vi "Refresh Players.vi"(11 "Dashboard":refnum<vi>) -> ()   [LabVIEW 2015, in "SB SubVIs.lvlib"]
uses:
  SB SubVIs.lvlib
  Type Defs/Dashboard.ctl
  Type Defs/Add Player.ctl
  Square/Square.lvclass
  Globals (private).vi
  Type Defs/SB Type Defs.lvlib
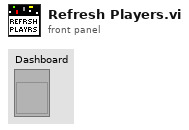
[diagram p1: front panel]
types:
  T1 = cluster{"Square out":refnum<class "Square.lvclass">, "Name":string, "Victory Speech":string}
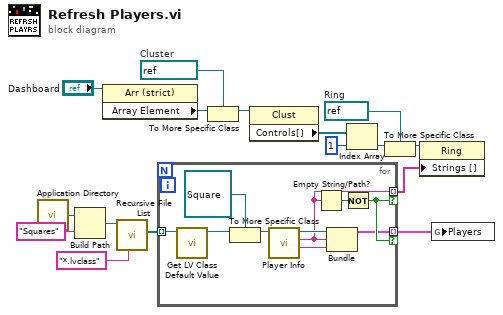
[diagram p0: block diagram]
diagram:
  w4 = refnum<vi> refnum  # Ring
  w9 = refnum<vi> refnum  # Cluster
  n1 = call <vilib>:"Application Directory.vi"() -> ("Application Directory"=w13:path)
  n2 = Build Path(base path=w13, name or relative path="Squares") -> (appended path=w11:path)
  n3 = property class="Arr (strict)"(reference="Dashboard") -> ("Array Element"=w10:refnum<vi>)  [unwired: 1 in, 2 out]
  n4 = call <vilib>:"Recursive File List.vi"("pattern"="*.lvclass", "Folder Path"=w11) -> ("All Files in Dir"=w15:path[])  [unwired: 5 in, 4 out]
  n5 = for {
    tunnel: w15 -> [w26] mode=indexing
    tunnel: [w18] -> w14 mode=indexing if=w20
    tunnel: [w19] -> w1 mode=indexing if=w20
    n6 = call <vilib>:"Get LV Class Default Value.vi"("class path"=w26) -> ("object"=w25:refnum<class>)  [unwired: 9 in, 1 out]
    n7 = To More Specific Class(target class=refnum<class "Square.lvclass"> refnum ("Runner.lvclass"), reference=w25) -> (specific class reference=w22:refnum<class "Square.lvclass">)  [unwired: 1 in, 1 out]
    n8 = call-dynamic "Player Info.vi"("Square in"=w22) -> ("Victory Speech"=w17:string, "Name"=w18:string, "Square out"=w21:refnum<class "Square.lvclass">)  [unwired: 8 in]
    n9 = Empty String/Path?(string/path=w18) -> (empty?=w23:bool)
    n10 = Bundle("Square out"=w21, "Name"=w18, "Victory Speech"=w17) -> (w19:T1)  [unwired: 1 in]
    n11 = Not(x=w23) -> (.not. x?=w20:bool)
  }
  n12 = To More Specific Class(target class=w9, reference=w10) -> (specific class reference=w8:refnum<vi>)  [unwired: 1 in, 1 out]
  n13 = property class="Clust"(reference=w8) -> ("Controls[]"=w7:refnum<vi>[])  [unwired: 1 in, 2 out]
  n14 = Index Array(array=w7, index=1) -> (element=w5:refnum<vi>)
  n15 = To More Specific Class(target class=w4, reference=w5) -> (specific class reference=w3:refnum<vi>)  [unwired: 1 in, 1 out]
  n16 = property on="Property Node" class="Ring"(reference=w3, "Strings []"=w14) -> ()  [unwired: 1 in, 2 out]
  n17 = global write "Globals (private).vi" "Players"(w1) -> ()
